vi "Untitled 1.vi"() -> ()   [LabVIEW 2016]
panel:
  in  "开始":bool
  out "Waveform Chart":dynamicdata(graph)
  out "心率测试":string
  out "心率":u32
  out "测试结果":string
  out "报警":bool
  out "正常":bool
  out "心率转盘":dbl(knob) scale=0.0..150.0 scale format="%#1.11g"
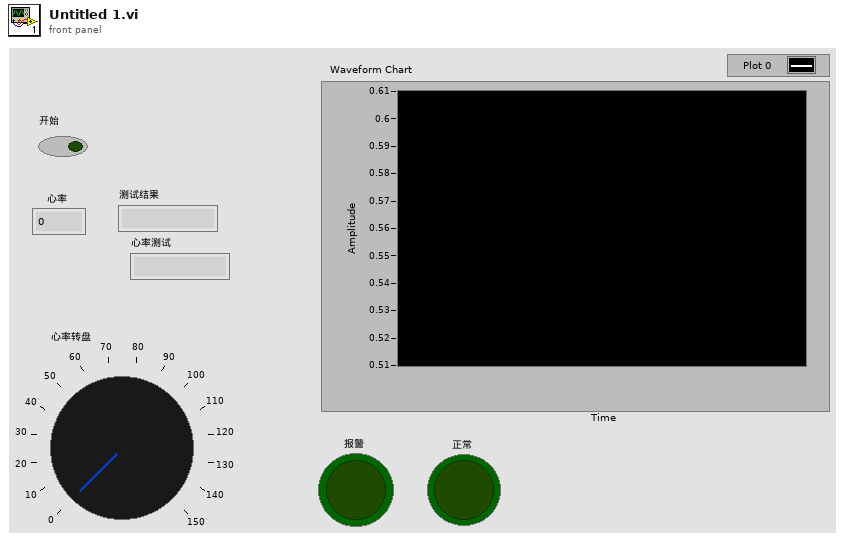
[diagram p1: front panel]
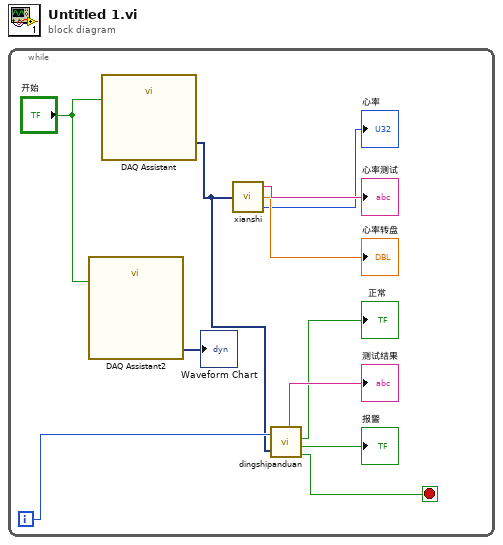
[diagram p0: block diagram]
diagram:
  n1 = while {
    i -> [w11]
    stop <- w7 stop-if-true
    n2 = call "DAQ Assistant2"("stop (T)"="开始") -> ("data"=→"Waveform Chart":dynamicdata)  [unwired: 16 in, 2 out]
    n3 = call "DAQ Assistant"("stop (F)"="开始") -> ("data"=w1:dynamicdata)  [unwired: 15 in, 3 out]
    n4 = call "xianshi.vi"("心率"=w1) -> ("标题"=→"心率测试":string, "心率转盘"=→"心率转盘":dbl, "心率"=→"心率":u32)
    n5 = call "dingshipanduan.vi"("i"=w11, "心率"=w1) -> ("测试结果"=→"测试结果":string, "正常"=→"正常":bool, "报警"=→"报警":bool, "开始"=w7:bool)
  }
